vi "_UserDialog Choose Driver ReadMe Params.vi"(0 "VI Default Path":path, 1 "LV <help> directory?":bool, 2 "Documentable VI Path":path, 11 "error in (no error)":errorcluster) -> (4 "HTML File Path":path, 14 "Cancelled by User?":bool, 15 "error out":errorcluster)   [LabVIEW 2012]
uses:
  _Controls and TypeDefs/UserDialogStates.ctl
  <vilib>/Platform/browser.llb/Open URL in Default Browser (string).vi
panel:
  in  "www.labicom.net":bool
  in  "Help Button":bool
  in  "Revision History":string="REV 1.0, 16/07/2012\nModified by: Igor Titov, Geneva, CERN.\nOriginal release." caption="Provide detailed driver revision history including driver revision number, date of revision, and description of revision made to driver"
  in  "IsKnownIssues? chkBox":bool=TRUE
  in  "KnownIssues":string
  in  "SupportEmail":string="instrument.drivers@ni.com"
  in  "RequiredSoftware":string="[VISA 3.0 or later]"
  in  "CurrentRevisionDate":string="15/08/2012"
  in  "OriginalReleaseDate":string="15/08/2012"
  in  "DriverRevision":string="1.0"
  in  "FirmwareTested":string="[8-5-12]"
  in  "Interfaces":string="[GPIB, Serial, USB, Ethernet]"
  in  "ModelsTested":string="[33120A, 33220A]"
  in  "Languages":string="[LabVIEW]"
  in  "Models":string="[33120A, 33220A, 33250A]"
  in  "Manufacturer":string="[Agilent]"
  in  "IsCodeAvailable? Combo":string(combo)="Yes"
  in  "IsSupported? Combo":string(combo)="No"
  in  "IsCertified? Combo":string(combo)="No"
  in  "ProjectStyleCombo":string(combo)="(project-style)"
  in  "Disclaimer":string="[Disclaimer text]"
  in  "IsDisclaimer? chkBox":bool=TRUE
  in  "Cancel Button":bool
  in  "GenerateReadme_btn":bool
  in  "Patents":string="[Patents text]"
  in  "Trademarks":string="[Trademarks text]"
  in  "Copyright":string="[Copyright text]"
  in  "Support CommunityForums":string=" [link to community forums or NI Community page and expected response time]"
  in  "SupportEmail":string="[Support email address and expected response time]"
  in  "SupportTelephone":string="[Telephone number and hours of operation]"
  in  "AppUpgrader":string="[Developer Name, Developer e-mail, Developer certification level (if any), Organization]"
  in  "AppDeveloper":string="[Developer Name, Developer e-mail, Developer certification level (if any), Organization]"
  out "Product Short Name 12":string="[DriverIdentifier]" caption="Product Short Name"
  in  "IsDeveloper? chkBox":bool=TRUE
  in  "Installation Instructions":string[][](table)=[["[Step 1]"], ["[Step 2]"]]
  out "Product Short Name 2":string="[DriverIdentifier]" caption="Driver Identifier"
  in  "IsCopyright? chkBox":bool=TRUE
  in  "IsPatents? chkBox":bool=TRUE
  in  "IsTrademarks? chkBox":bool=TRUE
  in  "IsContactSupport? chkBox":bool=TRUE
  in  "IsInstallation? chkBox":bool=TRUE
  in  "Year":string="[Year]"
  in  "Month":string="[Month]"
  in  "Driver Identifier":string="[Driver Identifier]"
  in  "Next_btn":bool
  # "Instrument Driver Readme"
  # "To rate this instrument driver, go the the driver download page on the Instrument Driver Network."
  # "The readme contains the following main sections:"
  # "Overview"
  # "Required software"
  # "Revision History"
  # "1. Overview"
  # "Instrument Driver Technology: LabVIEW Plug and Play"
  # "Manufacturer:"
  # "Supported Language(s):"
  # "Supported Model(s):"
  # "Model(s) Tested:"
  # "Interface(s):"
  # "Firmware Revision(s) Tested:"
  # "Certified:"
  # "NI Supported:"
  # "Source Code Available:"
  # "Driver Revision:"
  # "Original Release Date:"
  # "Current Revision Date:"
  # "2. Installation (if applicable)"
  # "This section documents installation instructions for"
  # "Instrument Driver."
  # "New line here corresponds to new item in the list in HTML"
  # "3. Required Software"
  # "Some software components need to be installed before using this instrument driver. \nThe minimum versions of these components are listed below."
  # "Refer to the LabVIEW Help for more information about software requirements. \nYou access the LabVIEW Help by selecting Help»Search the LabVIEW Help."
  # "4. Known Issues (if applicable)"
  # "To report issues or provide feedback about this instrument driver, please send an email to"
  # "Include instrument functionality not supported by the driver or known issues as necessary."
  # "5. Revision History"
  # "The latest version of this and other LabVIEW and LabWindows/CVI instrument drivers can be downloaded \nat the Instrument Driver Network."
  # "6. Developer(s) of"
  # "Instrument Driver"
  # "(if applicable)"
  # "Step 2/2:\nConfigure VI Documentation Layout"
  # "This instrument driver was \ndeveloped by"
  # "Additional layout elements for LabVIEW help"
  # "This icon denotes a note, which alerts you\nto important information. You can add it\nby placing <_note_> into your text."
  # "Caution: place <_caution_> into your text"
  # "Last upgrade of this instrument driver was made by"
  # "Note: place <_note_> into your text"
  # "This icon denotes a caution, which \nadvises you of precautions to take to \navoid injury, data loss, or a system crash.\nYou can add it by placing <_caution_>\ninto your text."
  # "Mandatory Fields"
  # "7. Contact Support"
  # "Tip: place <_tip_> into your text"
  # "(if applicable)"
  # "You can contact our support staff by one of the following:"
  # "Windows"
  # "Platform: enclose platform name between\n<_platform_> and </_platform_> tags"
  # "Text in blue color denotes a specific \nplatform and indicates that the text \nfollowing it applies only to that platform.\nYou can add it enclosing platform name\nbetween <_platform_> and </_platform_>\ntags (e.g.: <_platform_>MacOS X</_platform_>)."
  # "Telephone:"
  # "bold"
  # "Text in bold: enclose such text between\n<B> and </B> tags"
  # "Email:"
  # "Community Forums:"
  # "Attention!"
  # "Caution Text: enclose such text between \n<_caution_text_> and </_caution_text_> tags"
  # "Bold text denotes items that you must \nselect or click on in the software, such as \nmenu items and dialog box options. \nBold text also denotes parameter names, \nemphasis, or an introduction to a key \nconcept. You can emphasize such text by \nenclosing in between <B> and </B> tags."
  # "vigods.com"
  # "Link: place relative path in place of '_path_' and\ntext in place of '_text_' and insert resulting string\nwherever you need: \n<a href=\"_path_\">_text_</a>"
  # "8. Copyright"
  # "monospace"
  # "Monospace: enclose such text between\n<_monospace_> and </_monospace_> tags"
  # "(if applicable)"
  # "9. Trademarks"
  # "(if applicable)"
  # "10. Patents"
  # "(if applicable)"
  # "11. Disclaimer"
  # "(if applicable)"
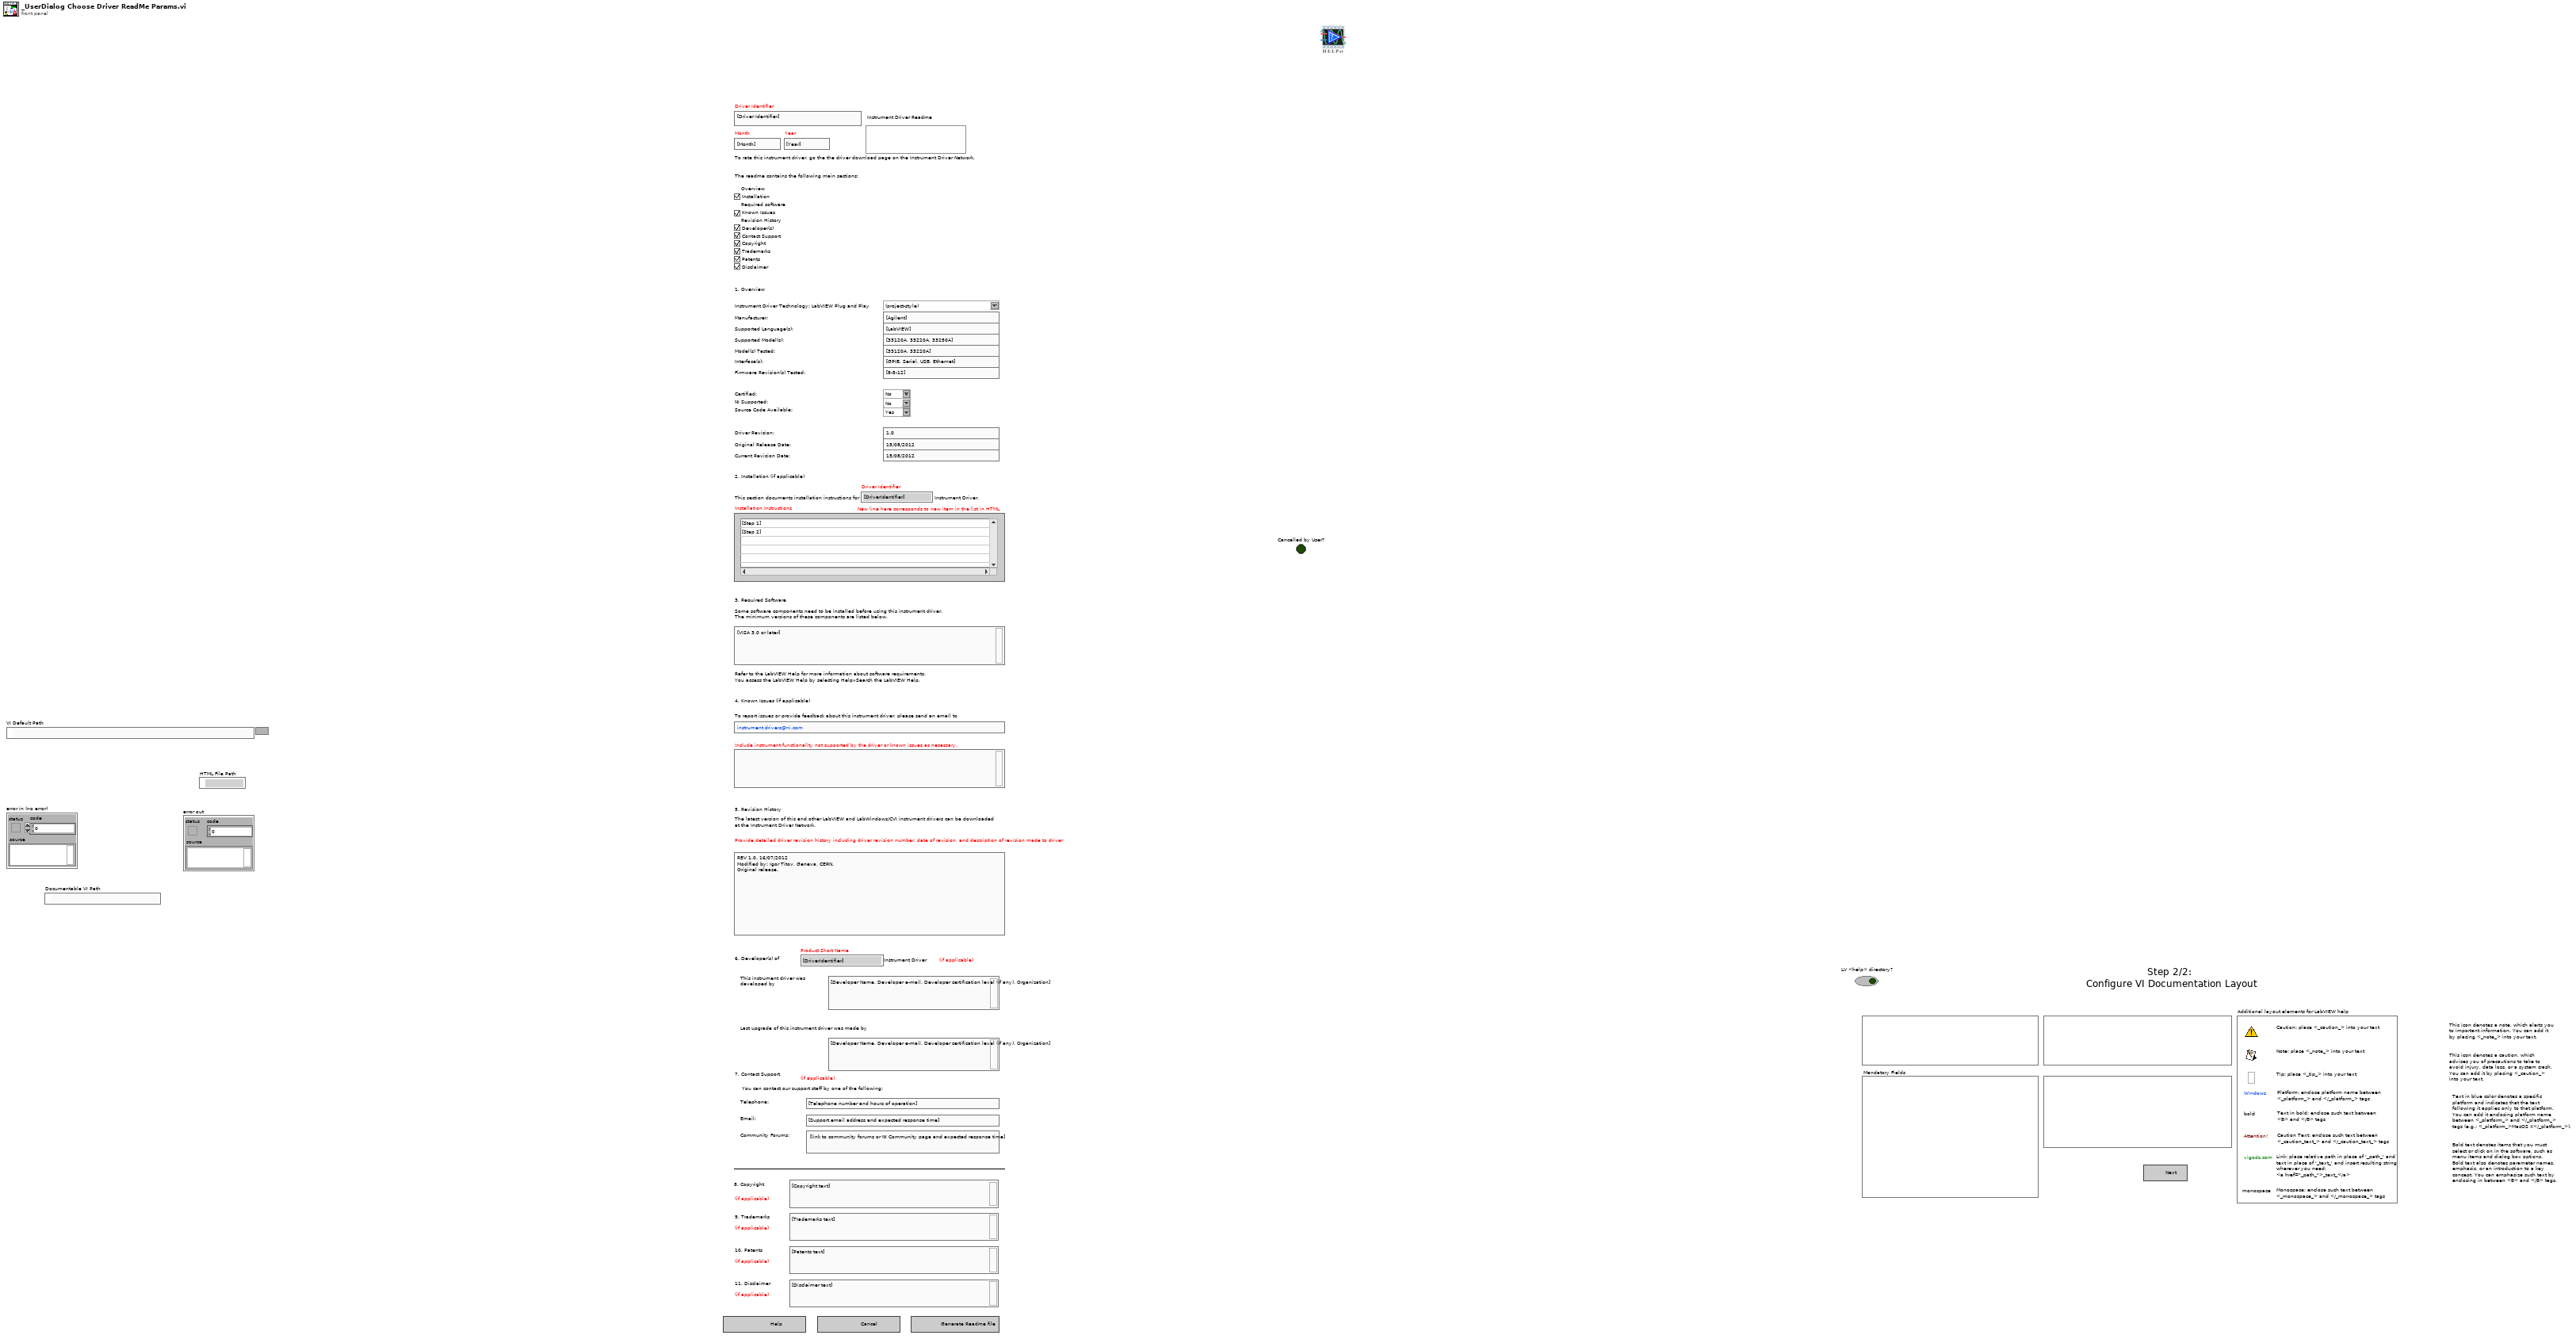
[diagram p1: front panel]
types:
  T1 = typedef "UserDialogStates.ctl" = enum16{"Overview", "Known Issues", "Choose parameters", "Update", "Choose HTML file path", "Choose Images directory path", "Decide if there is Context Help", "Choose help hierarchy", "Generate HTML", "Installation", "System Requirements", "Software Support", "Device Support", "Upgrade Issues", "New Features", "Fixed Issues", "Developer", "Contact Support", "Copyright", "Trademarks", "Patents", "Disclaimer", "Save", "Shutdown"}
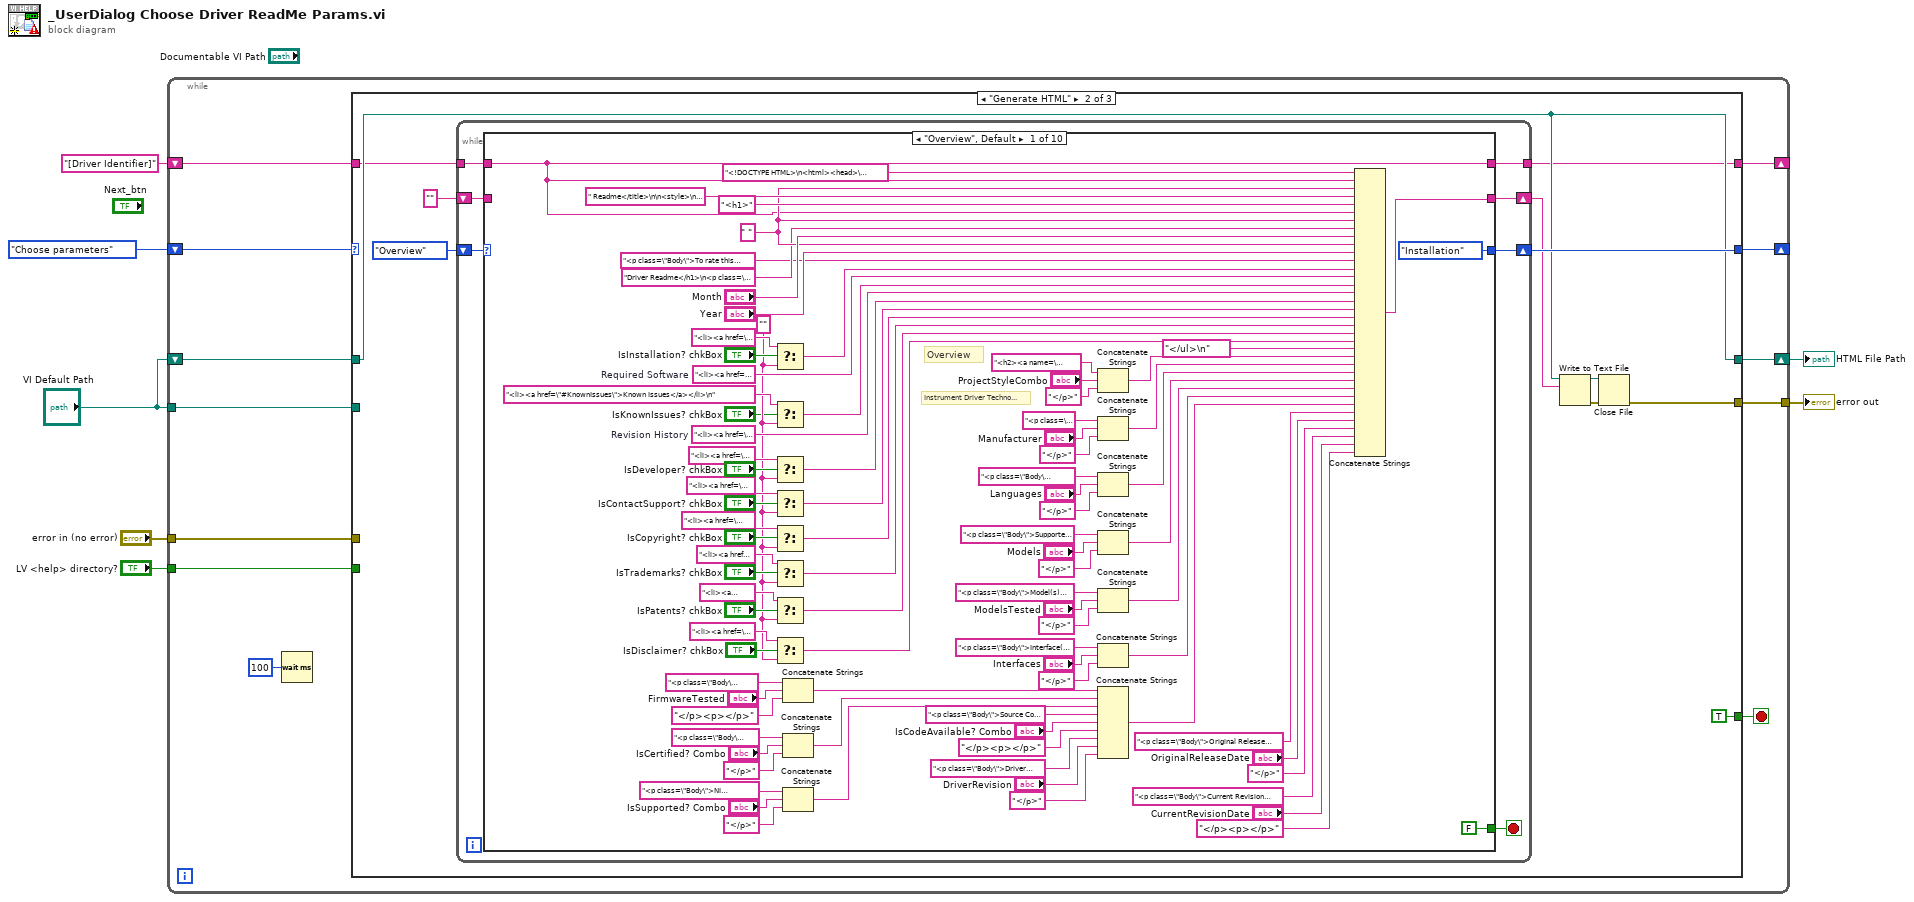
[diagram p0: block diagram]
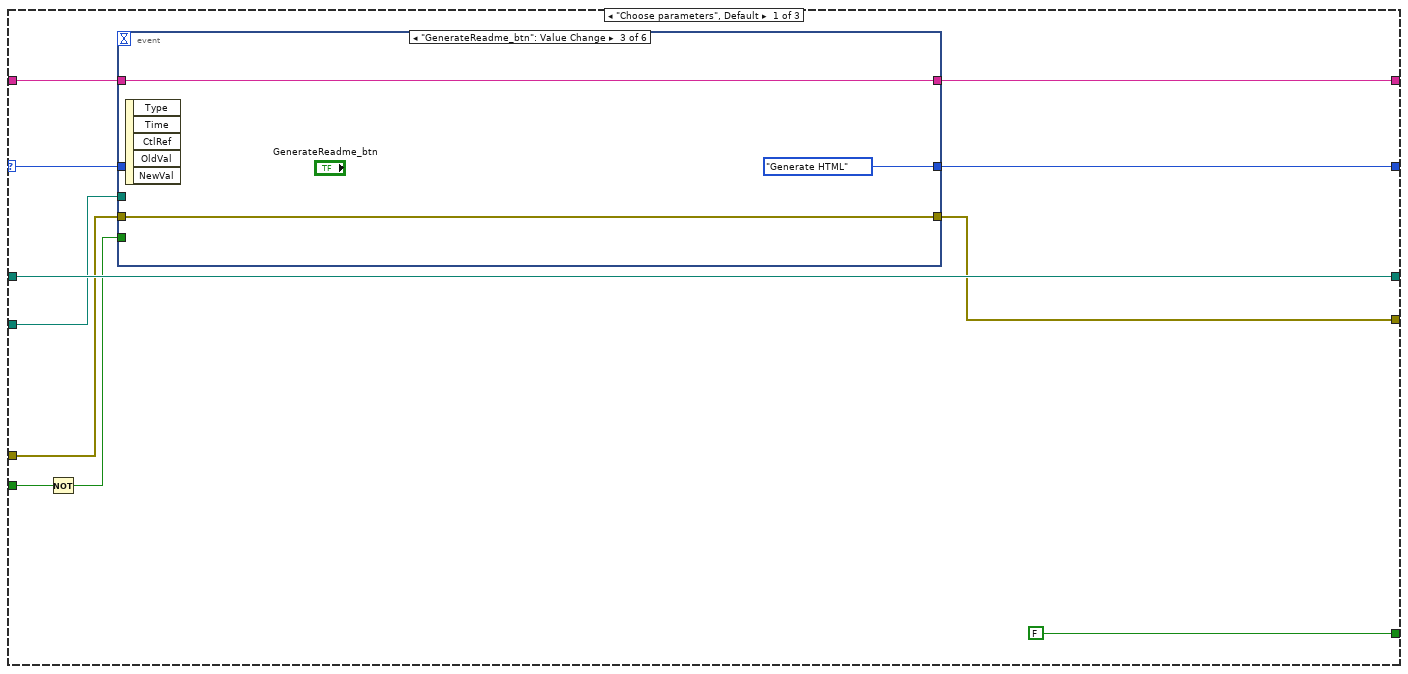
[diagram p2: hidden frame]
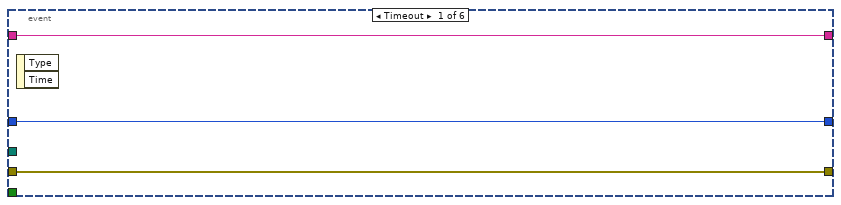
[diagram p3: hidden frame]
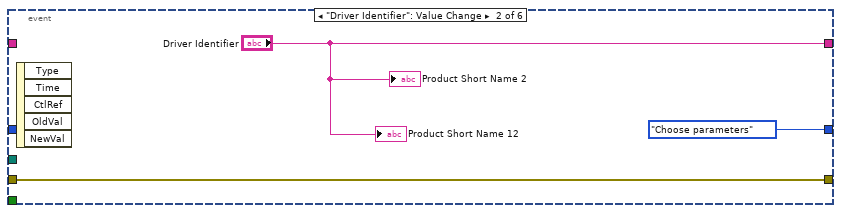
[diagram p4: hidden frame]
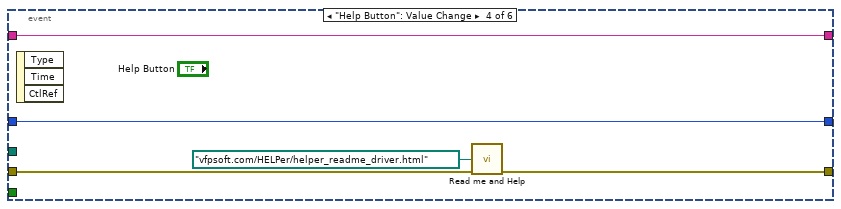
[diagram p5: hidden frame]
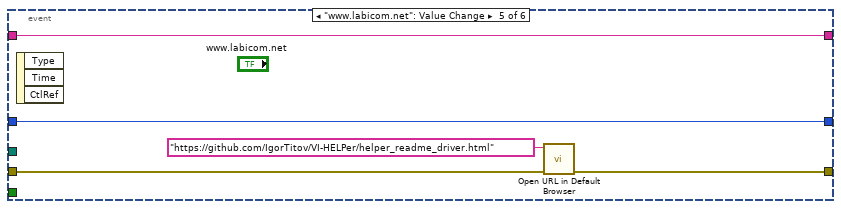
[diagram p6: hidden frame]
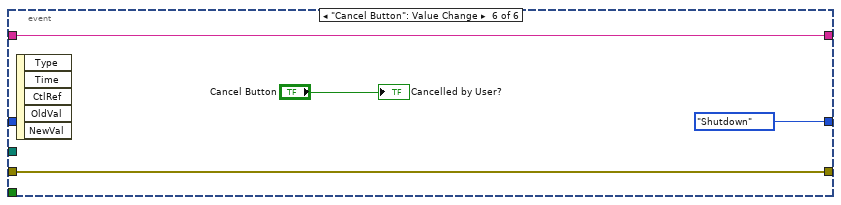
[diagram p7: hidden frame]
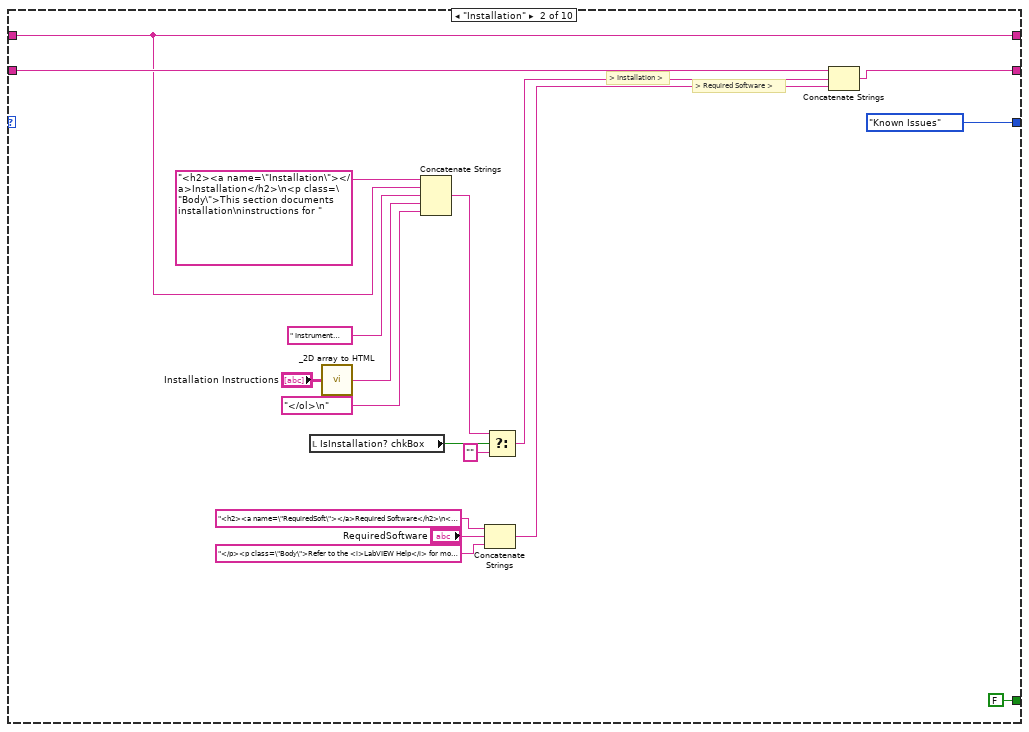
[diagram p8: hidden frame]
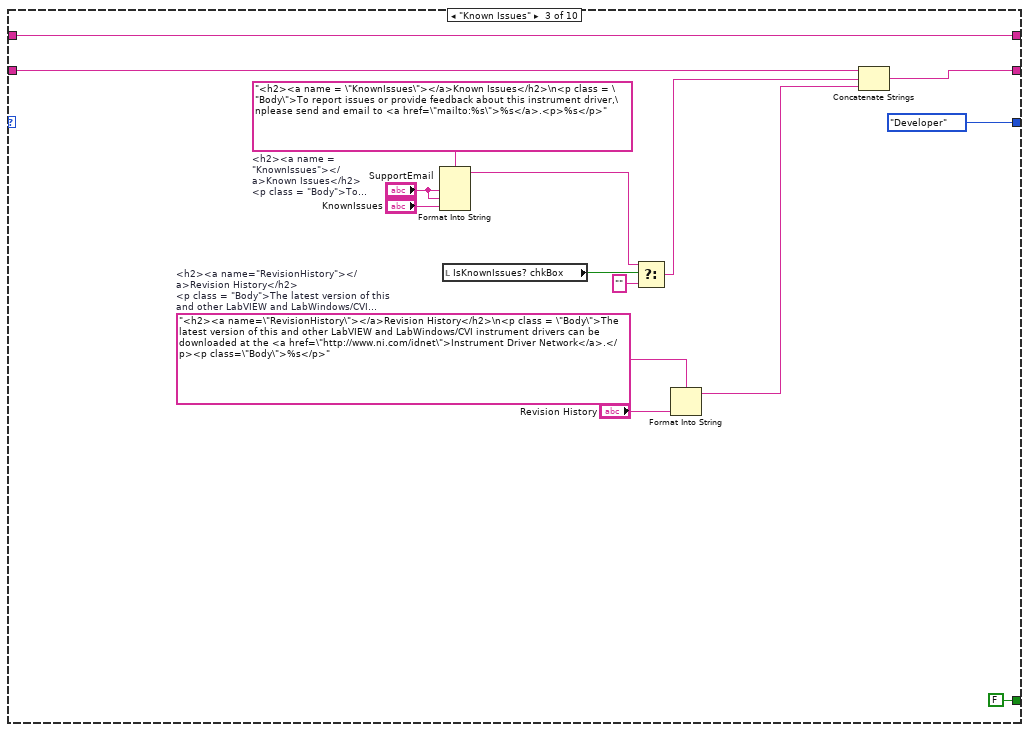
[diagram p9: hidden frame]
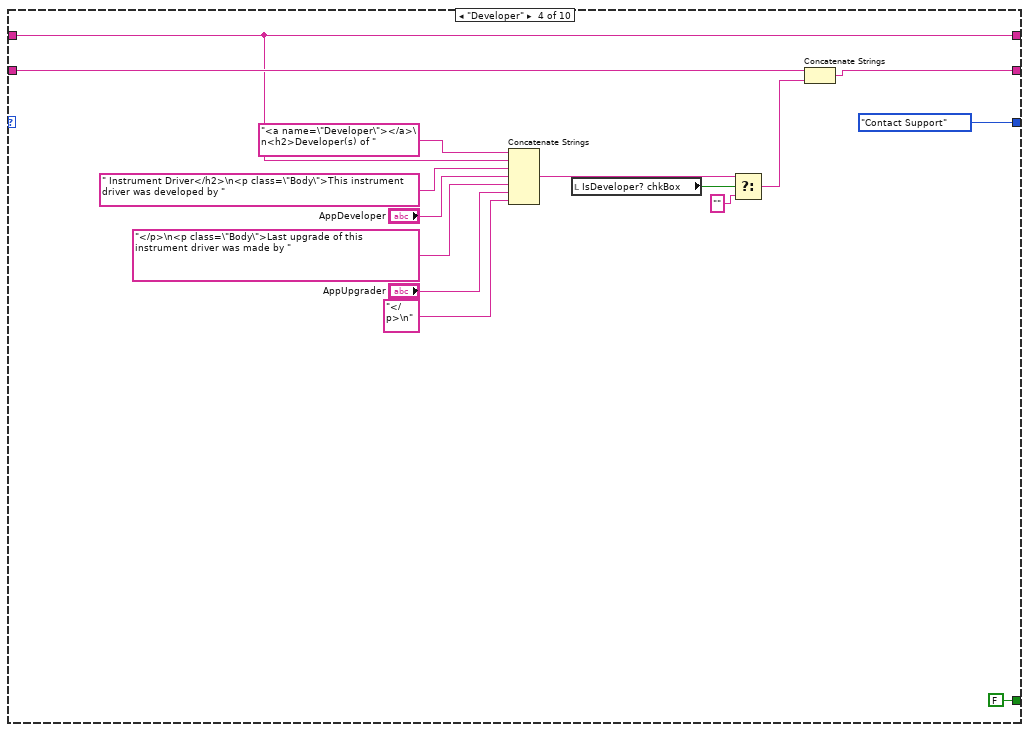
[diagram p10: hidden frame]
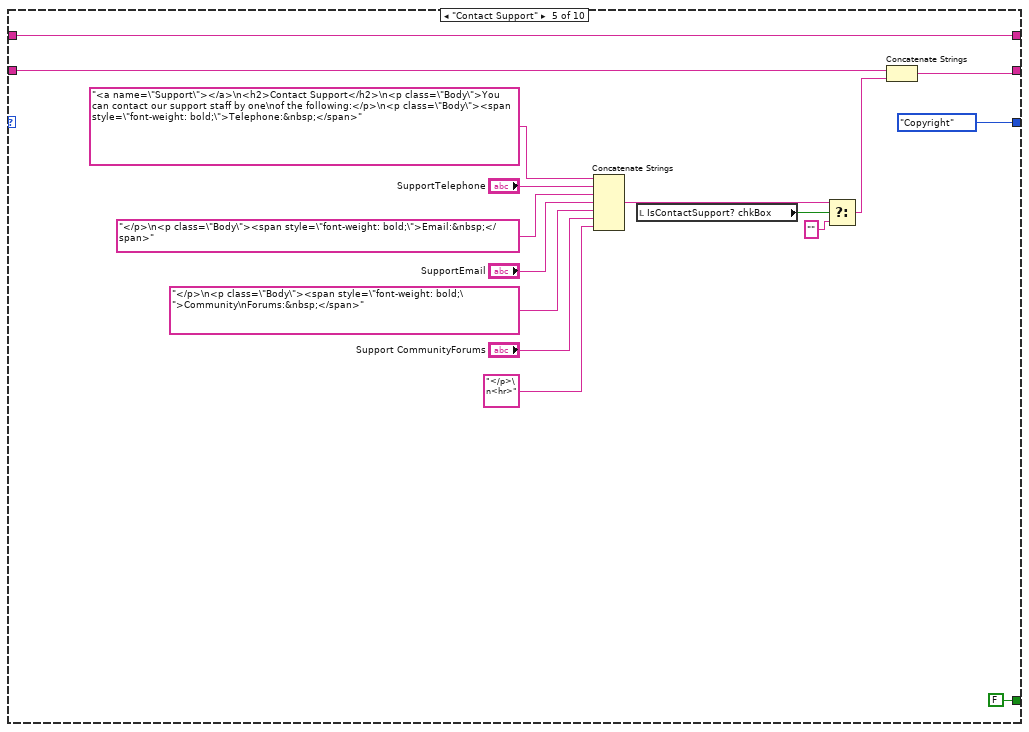
[diagram p11: hidden frame]
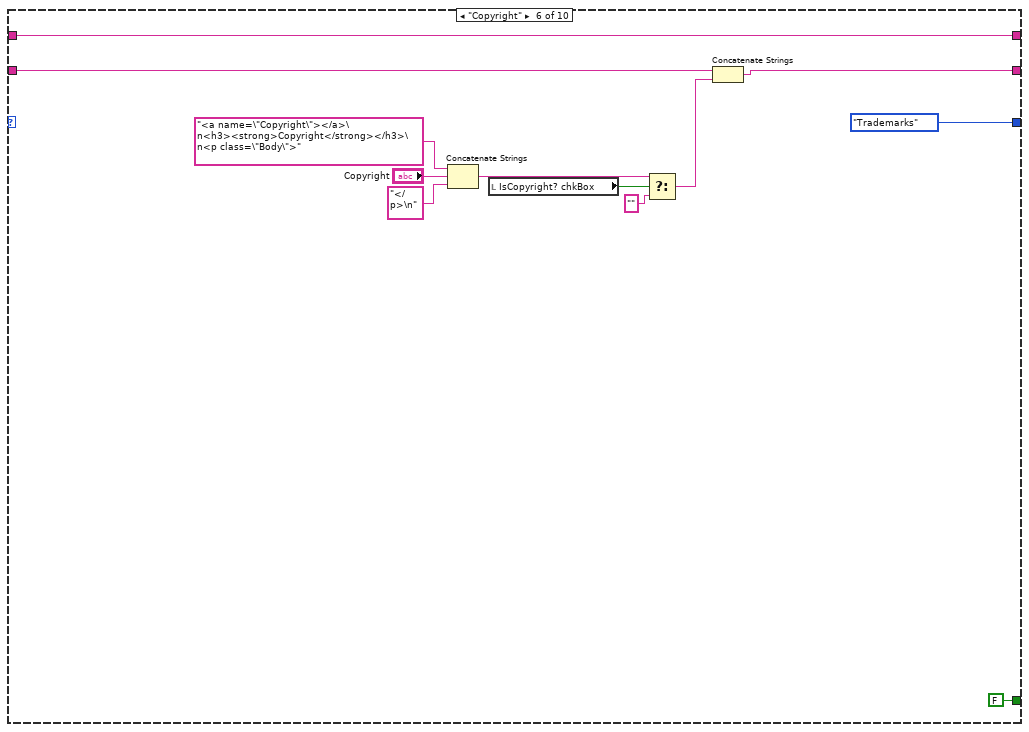
[diagram p12: hidden frame]
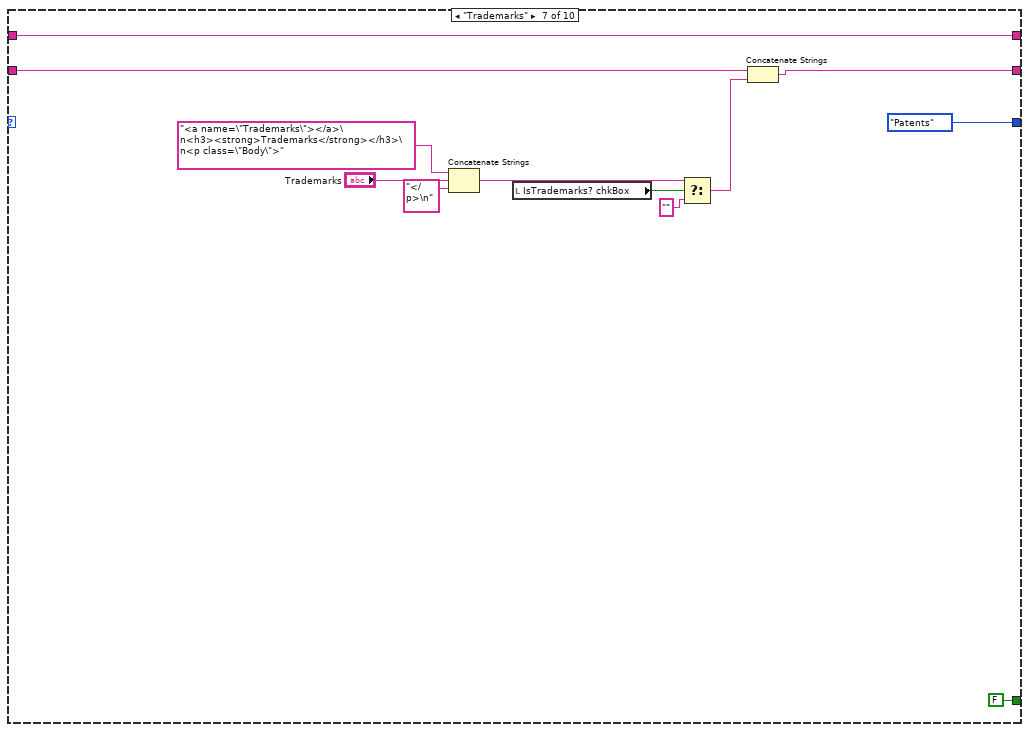
[diagram p13: hidden frame]
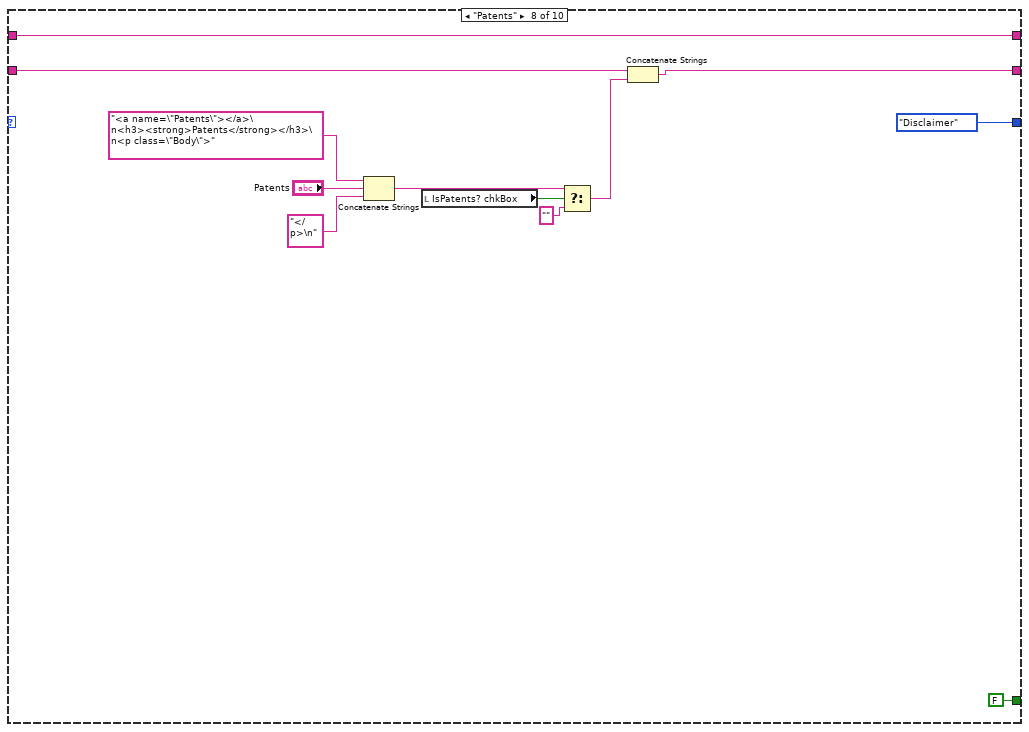
[diagram p14: hidden frame]
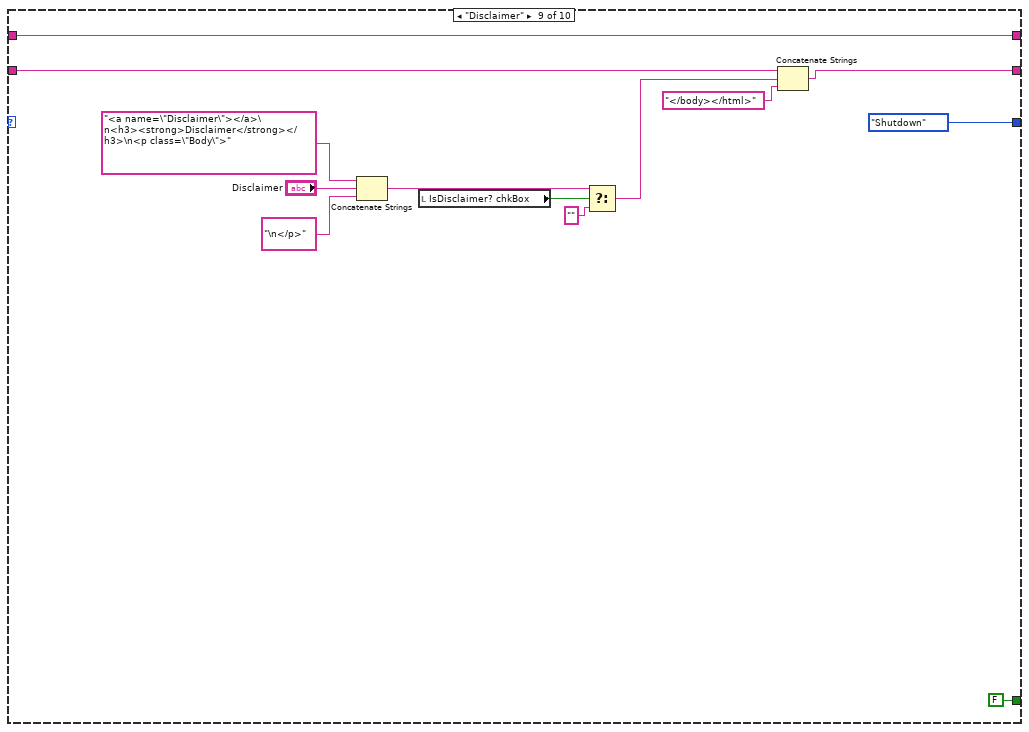
[diagram p15: hidden frame]
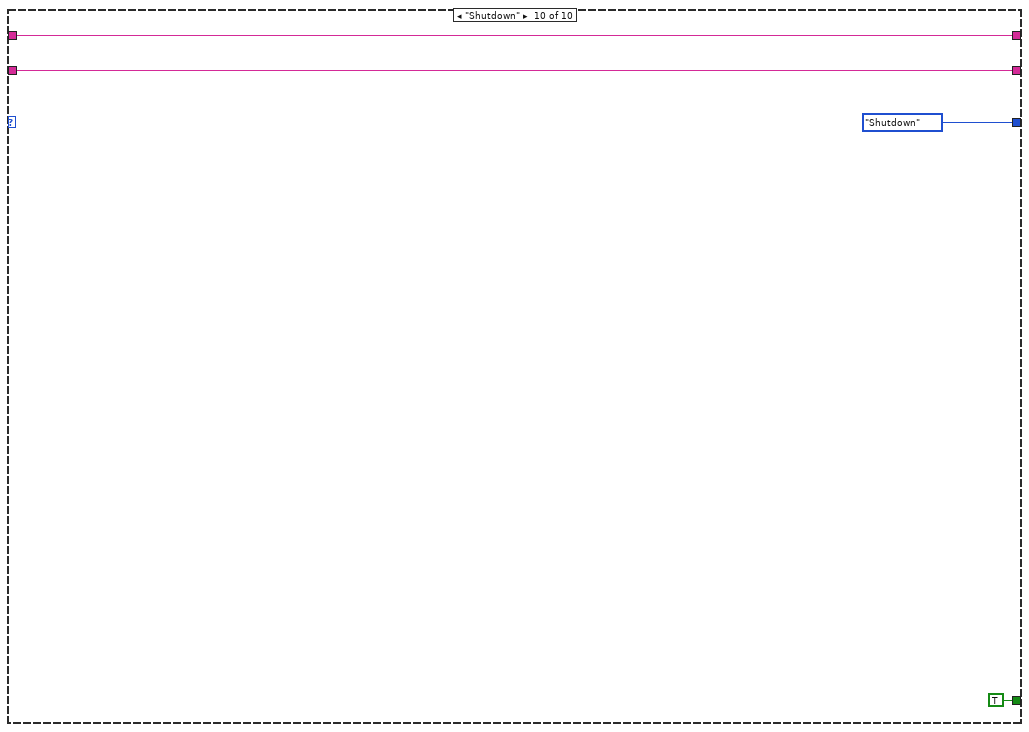
[diagram p16: hidden frame]
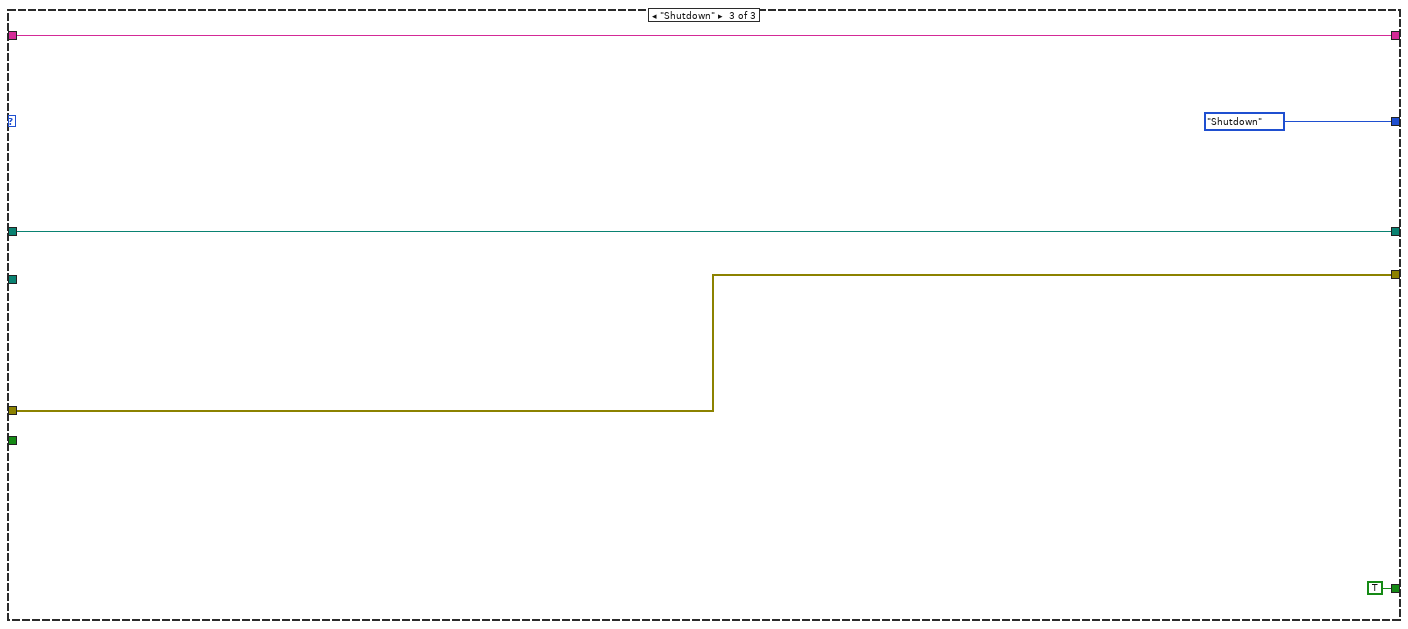
[diagram p17: hidden frame]
diagram:
  n1 = while {
    shift-right: [w16] -> _
    shift-left: UserDialogStates."Choose parameters" ("UserDialogSteps") -> [w17]
    tunnel: "VI Default Path" -> [w15]
    shift-right: [w14] -> w6
    shift-left: "VI Default Path" -> [w13]
    tunnel: "LV <help> directory?" -> [w8]
    tunnel: "error in (no error)" -> [w12]
    shift-right: [w11] -> _
    shift-left: "[Driver Identifier]" ("Driver Identifier") -> [w10]
    tunnel: [w9] -> w1
    stop <- w19 stop-if-true
    n2 = Wait (ms)(milliseconds to wait=u32 100) -> ()  [unwired: 1 out]
    n3 = case shown="\"Generate HTML\"" w17 {
      selector: w17 -> [w29 _ _]
      tunnel: [FALSE TRUE TRUE] -> w19
      tunnel: [w28 w63 UserDialogStates."Shutdown" ("UserDialogSteps")] -> w16
      tunnel: w15 -> [w25 _ _]
      tunnel: [w27 w61 w282] -> w14
      tunnel: w13 -> [w27 w61 w282]
      tunnel: w8 -> [w26 _ _]
      tunnel: w12 -> [w23 _ w278]
      tunnel: w10 -> [w22 w57 w280]
      tunnel: [w21 w56 w280] -> w11
      tunnel: [w20 w54 w278] -> w9
      frame "Choose parameters", Default {
        n4 = Not(x=w26) -> (.not. x?=w24:bool)
        n5 = event shown="[2] \"GenerateReadme_btn\": Value Change" {
          selector: _ -> [_ _ _ _ _ _]
          dyn-events: _ -> [_ _ _ _ _ _]
          timeout: _ -> [_ _ _ _ _ _]
          tunnel: w29 -> [w33 _ _ w44 w45 _]
          tunnel: [w33 UserDialogStates."Choose parameters" ("UserDialogSteps") UserDialogStates."Generate HTML" ("UserDialogSteps") w44 w45 UserDialogStates."Shutdown" ("UserDialogSteps")] -> w28
          tunnel: w25 -> [_ _ _ _ _ _]
          tunnel: w24 -> [_ _ _ _ _ _]
          tunnel: w23 -> [w31 w35 w38 w42 w48 w51]
          tunnel: w22 -> [w32 _ w39 w43 w46 w52]
          tunnel: [w32 "Driver Identifier" w39 w43 w46 w52] -> w21
          tunnel: [w31 w35 w38 w41 w47 w51] -> w20
          event Timeout {
            n6 = event-data() -> ()  [unwired: 1 in, 2 out]
          }
          event "Driver Identifier": Value Change {
            n7 = event-data() -> ()  [unwired: 1 in, 5 out]
            "Product Short Name 2" <- "Driver Identifier"
            "Product Short Name 12" <- "Driver Identifier"
          }
          event "GenerateReadme_btn": Value Change {
            n8 = event-data() -> ()  [unwired: 1 in, 5 out]
          }
          event "Help Button": Value Change {
            n9 = event-data() -> ()  [unwired: 1 in, 3 out]
            n10 = call "Read me and Help.vi"("path"=path "vfpsoft.com/HELPer/helper_readme_driver.html", "error in"=w42) -> ("error out"=w41:errorcluster)  [unwired: 13 in]
          }
          event "www.labicom.net": Value Change {
            n11 = event-data() -> ()  [unwired: 1 in, 3 out]
            n12 = call-poly <vilib>:"Open URL in Default Browser.vi"("error in (no error)"=w48, "URL"="https://github.com/IgorTitov/VI-HELPer/helper_readme_driver.html") -> ("error out"=w47:errorcluster)  [unwired: 4 in, 1 out]
          }
          event "Cancel Button": Value Change {
            n13 = event-data() -> ()  [unwired: 1 in, 5 out]
            "Cancelled by User?" <- "Cancel Button"
          }
        }
      }
      frame "Generate HTML" {
        n14 = while {
          shift-right: [w70] -> w63
          shift-left: UserDialogStates."Overview" ("UserDialogSteps") -> [w71]
          shift-right: [w68] -> w60
          shift-left: "" -> [w69]
          tunnel: w57 -> [w66]
          tunnel: [w65] -> w56
          stop <- w67 stop-if-true
          n15 = case shown="\"Overview\", Default" w71 {
            tunnel: [UserDialogStates."Installation" ("UserDialogSteps") UserDialogStates."Known Issues" ("UserDialogSteps") UserDialogStates."Developer" ("UserDialogSteps") UserDialogStates."Contact Support" ("UserDialogSteps") UserDialogStates."Copyright" ("UserDialogSteps") UserDialogStates."Trademarks" ("UserDialogSteps") UserDialogStates."Patents" ("UserDialogSteps") UserDialogStates."Disclaimer" ("UserDialogSteps") UserDialogStates."Shutdown" ("UserDialogSteps") UserDialogStates."Shutdown" ("UserDialogSteps")] -> w70
            tunnel: w69 -> [_ w169 w191 w206 w221 w233 w245 w257 w269 w276]
            tunnel: [w124 w167 w190 w205 w220 w232 w244 w256 w271 w276] -> w68
            tunnel: [FALSE FALSE FALSE FALSE FALSE FALSE FALSE FALSE FALSE TRUE] -> w67
            tunnel: w66 -> [w73 w162 w187 w195 w210 w226 w238 w250 w262 w275]
            tunnel: [w73 w162 w187 w195 w210 w226 w238 w250 w262 w275] -> w65
            frame "Overview", Default {
              w126 = "<li><a href=\"#RevisionHistory\">Revision History</a></li>\n"  # Revision History
              w127 = "<li><a href=\"#RequiredSoft\">Required Software</a></li>\n"  # Required Software
              w125 = ""
              w130 = " " ("string")
              # "Instrument Driver Techno..."
              # "Overview"
              n16 = Select(t="<li><a href=\"#Installation\">Installation</a></li>\n", s="IsInstallation? chkBox", f=w125) -> (s? t:f=w156:string)
              n17 = Select(t="<li><a href=\"#KnownIssues\">Known Issues</a></li>\n", s="IsKnownIssues? chkBox", f=w125) -> (s? t:f=w154:string)
              n18 = Select(t="<li><a href=\"#Developer\">Developer(s)</a></li>", s="IsDeveloper? chkBox", f=w125) -> (s? t:f=w152:string)
              n19 = Select(t="<li><a href=\"#Support\">Contact Support</a></li>\n", s="IsContactSupport? chkBox", f=w125) -> (s? t:f=w149:string)
              n20 = Select(t="<li><a href=\"#Copyright\">Copyright</a></li>\n", s="IsCopyright? chkBox", f=w125) -> (s? t:f=w145:string)
              n21 = Select(t="<li><a href=\"#Trademarks\">Trademarks</a></li>\n", s="IsTrademarks? chkBox", f=w125) -> (s? t:f=w139:string)
              n22 = Select(t="<li><a href=\"#Patents\">Patents</a></li>\n", s="IsPatents? chkBox", f=w125) -> (s? t:f=w138:string)
              n23 = Select(t="<li><a href=\"#Disclaimer\">Disclaimer</a></li>\n", s="IsDisclaimer? chkBox", f=w125) -> (s? t:f=w135:string)
              n24 = Concatenate Strings("<p class=\"Body\">Firmware Revision(s) Tested: ", "FirmwareTested", "</p><p></p>") -> (w88:string)
              n25 = Concatenate Strings("<p class=\"Body\">Certified: ", "IsCertified? Combo", "</p>") -> (w87:string)
              n26 = Concatenate Strings("<p class=\"Body\">NI Supported: ", "IsSupported? Combo", "</p>") -> (w86:string)
              n27 = Concatenate Strings("<h2><a name=\"Overview\"></a>Overview</h2>\n<p class=\"Body\">Instrument Driver Technology: LabVIEW Plug and Play ", "ProjectStyleCombo", "</p>") -> (w121:string)
              n28 = Concatenate Strings("<p class=\"Body\">Manufacturer: ", "Manufacturer", "</p>") -> (w117:string)
              n29 = Concatenate Strings("<p class=\"Body\">Supported Language(s): ", "Languages", "</p>") -> (w113:string)
              n30 = Concatenate Strings("<p class=\"Body\">Supported Model(s): ", "Models", "</p>") -> (w109:string)
              n31 = Concatenate Strings("<p class=\"Body\">Model(s) Tested: ", "ModelsTested", "</p>") -> (w105:string)
              n32 = Concatenate Strings("<p class=\"Body\">Interface(s): ", "Interfaces", "</p>") -> (w101:string)
              n33 = Concatenate Strings(w88, w87, w86, "<p class=\"Body\">Source Code Available: ", "IsCodeAvailable? Combo", "</p><p></p>", "<p class=\"Body\">Driver Revision: ", "DriverRevision", "</p>") -> (w85:string)
              n34 = Concatenate Strings("<!DOCTYPE HTML>\n<html><head>\n<meta http-equiv=\"Content-Type\" content=\"text/html; charset=ISO-8859-1\">\n<META NAME=\"GENERATOR\" CONTENT=\"HELPer - VI Documentation Toolkit from https://github.com/IgorTitov/VI-HELPer\">\n<script>\nfunction Link(URL)\n{\nwindow.location = URL;\n}\n</script>\n<meta http-equiv=\"Content-Type\" content=\"text/html; charset=ISO-8859-1\"><title>", w73, w130, " Readme</title>\n\n<style>\n/***************************************************/\n/* MINIMAL STYLES */\n/* The following section defines styles that every HTML Help project should\nneed. */\n/* The default style of P is red to alert you that you need to apply a style\nclass, such as Body. */\nP { margin-top:6.00pt; margin-bottom:6.00pt; font-family:Verdana; font-size:8pt;\ncolor: #FF0000; }\nBR { font-size:4.00pt; }\n/* Use H1 for all topic headings. */\nH1 { margin-top:3.00pt; margin-bottom:3.00pt; font-family:Verdana;\nfont-size:12pt; font-weight:bold; }\n/* Use H2 for second-level headings. */\nH2 { margin-top:9.00pt; margin-bottom:3.00pt; font-family:Verdana;\nfont-size:10pt; font-weight:bold; }\n/* Use H3 for third-level headings. */\nH3 { margin-top:6.00pt; margin-bottom:3.00pt; font-family:Verdana;\nfont-size:8pt; font-weight:bold; }\n/* Use H4 for fourth-level headings. */\nH4 { margin-top:3.00pt; margin-bottom:3.00pt; font-family:Verdana;\nfont-size:8pt; font-weight:bold; }\n/* H5 and H6 have the same definition as H4 because you should not need this\nlevel of heading in one topic. If you need to use H5 or H6, consider breaking up\nyour topic into more than one topic. */\nH5 { margin-top:3.00pt; margin-bottom:3.00pt; font-family:Verdana;\nfont-size:8pt; font-weight:bold; }\nH6 { margin-top:3.00pt; margin-bottom:3.00pt; font-family:Verdana;\nfont-size:8pt; font-weight:bold; }\n/* Use the Body style class for normal paragraphs. */\nP.Body { margin-top:6.00pt; margin-bottom:6.00pt; font-family:Verdana;\nfont-size:8pt; color:black; }\n/* Use the Anchor style class for graphic references on a line by themselves. */\nP.Anchor { margin-top:6.00pt; margin-bottom:6.00pt; font-family:Verdana;\nfont-size:10pt; color:black; }\n/* Use the Indent style classes to indent a paragraph. If you need to indent\ntext below a list item, use <br><br> to start the new paragraph within the same\nset of <li></li> tags. If you need to indent a list within another list, nest\nthe indented list within the first list's set of <ol></ol> or <ul></ul> tags. */\nP.Indent1 { margin-left:12.00pt; margin-top:6.00pt; margin-bottom:3.00pt;\nfont-family:Verdana; font-size:8pt; color:black; }\nP.Indent2 { margin-left:24.00pt; margin-top:6.00pt; margin-bottom:3.00pt;\nfont-family:Verdana; font-size:8pt; color:black; }\nP.Indent3 { margin-left:36.00pt; margin-top:6.00pt; margin-bottom:3.00pt;\nfont-family:Verdana; font-size:8pt; color:black; }\n/* Use the LI style for all list items. */\nLI { margin-top:3.00pt; margin-bottom:3.00pt; font-family:Verdana;\nfont-size:8pt; color:black; }\n/* Use the OL style for numbered lists. You do not have to type the number for\neach list item in a numbered list. */\nOL { margin-left:18.00pt; margin-top:3.00pt; margin-bottom:3.00pt;\ntext-indent:0pt; font-family:Verdana; font-size:8pt; color:black;\nlist-style-type: decimal; }\n/* Use the EquationNum style class for numbered lists of equations. You do not\nhave to type the number for each list item in a numbered list. */\nOL.EquationNum { margin-left:36.00pt; margin-top:3.00pt; margin-bottom:3.00pt;\ntext-indent:0pt; font-family:Verdana; font-size:8pt; color:black;\nlist-style-type: decimal; }\n/* Use the List-abc style class for lettered lists. You do not have to type the\nletter for each list item in a lettered list. */\nOL.List-abc { margin-left:18.00pt; margin-top:3.00pt; margin-bottom:3.00pt;\ntext-indent:0pt; font-family:Verdana; font-size:8pt; color:black;\nlist-style-type:lower-alpha; }\n/* Use the UL style for bulleted lists. You do not have to type the bullet for\neach list item in a bulleted list. */\nUL { margin-left:12.00pt; text-indent:0pt; margin-top:3.00pt;\nmargin-bottom:3.00pt; font-family:Verdana; font-size:8pt; color:black;\nlist-style-type: disc; }\n/* Use the List-Box style class for bulleted lists with boxes instead of\nbullets. You do not have to type the box for each list item in a box list. */\nUL.List-Box { margin-left:12.00pt; margin-top:3.00pt; margin-bottom:3.00pt;\ntext-indent:0pt; font-family:Verdana; font-size:8pt; color:black;\nlist-style-type: square; }\n/* Use the List-Diamond style class for bulleted lists with diamonds instead of\nbullets. You do not have to type the diamond for each list item in a diamond\nlist. */\nUL.List-Diamond { margin-left:12.00pt; margin-top:3.00pt; margin-bottom:3.00pt;\ntext-indent:0pt; font-family:Verdana; font-size:8pt; color:black;\nlist-style-image:url(diamond.gif); }\n/* Use the List-Hyphen style class for bulleted lists with hyphens instead of\nbullets. You do not have to type the hyphen for each list item in a hyphen list.\n*/\nUL.List-Hyphen { margin-left:12.00pt; margin-top:3.00pt; margin-bottom:3.00pt;\ntext-indent:0pt; font-family:Verdana; font-size:8pt; color:black;\nlist-style-image:url(hyphen.gif); }\n/* Use the Borderless style class for tables that do not need borders, such as\nfor 2-column or 3-column lists with no headings. */\nTable.Borderless { border:none; }\n/* Use the Bordered style class for tables that need borders. */\nTable.Bordered { border-width: 1pt; border-style: solid; border-color: black;\nborder-collapse: collapse; }\n/* Use the Borderless-Wide style class for tables that do not need borders and\nthat you want to stretch to fill the entire topic width. */\nTable.Borderless-Wide { border:none; width:100%; }\n/* Use the Bordered-Wide style class for tables that need borders and that you\nwant to stretch to fill the entire topic width. */\nTable.Bordered-Wide { border-width: 1pt; border-style: solid; border-color:\nblack; width:100%; border-collapse: collapse; }\n/* Use the TD style for table cells in Borderless or Borderless-Wide tables. */\nTD { font-family:Verdana; font-size:8pt; color:black; vertical-align:top;\npadding:3px; }\n/* Use the Bordered style class for table cells in Bordered or Bordered-Wide\ntables. */\nTD.Bordered { font-family:Verdana; font-size:8pt; color:black;\nvertical-align:top; border-width: 1pt; border-style: solid; border-color: black;\n}\n/* Use the Icon style class for table cells that contain note, caution, warning,\nor tip icons, or LabVIEW datatype terminals. */\nTD.Icon { width:40px; vertical-align:top; }\n/* Use the Table-cell-8pt style class for table cells in tables that contain a\nlot of information and need smaller text to fit it all on one screen to prevent\na horizontal scroll bar from appearing. */\nTD.Table-cell-8pt { font-family:Verdana; font-size:7pt; color:black; }\n/* Use the TH style for table heading cells in Borderless or Borderless-Wide\ntables. */\nTH { font-family:Verdana; font-size:8pt; color:black; font-weight:bold;\npadding:3px; }\n/* Use the Bordered style class for table heading cells in Bordered or\nBordered-Wide tables. */\nTH.Bordered { font-family:Verdana; font-size:8pt; color:black; font-weight:bold;\nborder-width: 1pt; border-style: solid; border-color: black; }\n/* Use the Table-cell-8pt style class for table heading cells in tables that\ncontain a lot of information and need smaller text to fit it all on one screen\nto prevent a horizontal scroll bar from appearing. */\nTH.Table-Head-8pt { font-family:Verdana; font-size:7pt; color:black;\nfont-weight:bold; }\n/* Use the Left-Align style class for table heading cells that you want to left\nalign instead of center align. */\nTH.Left-Align { font-family:Verdana; font-size:8pt; color:black;\nfont-weight:bold; padding:3px; text-align:left; }\n/***************************************************/\n/* CHARACTER FORMATS */\n/* The following section defines character formats that every HTML Help project\nshould need. */\n/* Use the Dark-Red format for warnings or cautions. */\n#Dark-Red { color: #800000 }\n/* Use the Monospace format for code or syntax examples. */\n#Monospace { font-family: Courier New; font-size: 8pt; }\n/* Use the Monospace-Bold format for messages and responses that the computer\nautomatically prints to the screen. */\n#Monospace-Bold { font-family: Courier New; font-size: 8pt; font-weight: bold; }\n/* Use the Monospace-Italic format to denote text that is a placeholder for a\nword or value that the user must supply. */\n#Monospace-Italic { font-family: Courier New; font-size: 8pt; font-style:\nitalic; }\n/* Use the Platform format to denote a specific platform. */\n#Platform { color: #0000FF; font-weight: bold; }\n/* Use the Symbol format for characters not in the Verdana character set. Use\nthis format sparingly. When possible, you should use the correct ASCII code for\nthe symbol or use a graphic to recreate the symbol. */\n#Symbol { font-family: Symbol; font-size: 8pt; }\n/* CHARACTER FORMATS Updated to conform with the CSE HTML Validator Pro */\n/* The following section defines character formats that every HTML Help project\nshould need. */\n/* Use the Dark-Red format for warnings or cautions. */\n.Dark-Red { color: #800000 }\n/* Use the Monospace format for code or syntax examples. */\n.Monospace { font-family: Courier New; font-size: 8pt; }\n/* Use the Monospace-Bold format for messages and responses that the computer\nautomatically prints to the screen. */\n.Monospace-Bold { font-family: Courier New; font-size: 8pt; font-weight: bold; }\n/* Use the Monospace-Italic format to denote text that is a placeholder for a\nword or value that the user must supply. */\n.Monospace-Italic { font-family: Courier New; font-size: 8pt; font-style:\nitalic; }\n/* Use the Platform format to denote a specific platform. */\n.Platform { color: #0000FF; font-weight: bold; }\n/* Use the Symbol format for characters not in the Verdana character set. Use\nthis format sparingly. When possible, you should use the correct ASCII code for\nthe symbol or use a graphic to recreate the symbol. */\n.Symbol { font-family: Symbol; font-size: 8pt; }\n/* Use the Red-text format to call attention to text that needs information\nadded or edited by techcomm */\n.Red-text {color: #FF0000;}\n/* Use the Green-Underline format for the green defintion in the conventions\ntopic */\n.Green-Underline {color: #007700; text-decoration : underline;}\n/* Use the glossButton format for the glossary buttons used in the glossary\ntopic */\n.glossButton { font-family:Verdana, sans-serif; font-size:12px; color:black; }\n/* Use for text sections and hyphenated words that should not break at line\nwraps */\nspan.nobreak{white-space:nowrap}\n/* The following styles define the color of links. */\na:link { color: #007700 }\na:hover { color: #FF0000 }\na:active { color: #FF0000 }\na:visited { color: #7F007F }\n/***************************************************/\n/* ACTIVITY STYLES */\n/* The following section defines styles that only tutorial-style HTML Help\nprojects should need. */\n/* Use the Activity-Objective style class for the objective at the beginning of\nan activity topic. */\nH3.Activity-Objective { color: #800000; }\n/***************************************************/\n/* CODE STYLES */\n/* The following section defines styles that you need to format entire sections\nof code or syntax examples. If you have just a few words you need to format as a\ncode or syntax example, use the Monospace character format. */\nP.Code { margin-top:3.00pt; margin-bottom:0.00pt; font-family:Courier New;\nfont-size:8pt; color:black; }\nP.Code1 { margin-left:12.00pt; margin-top:3.00pt; margin-bottom:0.00pt;\nfont-family:Courier New; font-size:8pt; color:black; }\nP.Code2 { margin-left:24.00pt; margin-top:3.00pt; margin-bottom:0.00pt;\nfont-family:Courier New; font-size:8pt; color:black; }\nP.Code3 { margin-left:36.00pt; margin-top:3.00pt; margin-bottom:0.00pt;\nfont-family:Courier New; font-size:8pt; color:black; }\n/***************************************************/\n/* FUNCTION STYLES */\n/* The following section defines styles that you might need to format function\nreference help. */\nP.F-VI-Code4 { margin-left:48.00pt; margin-top:3.00pt; margin-bottom:0.00pt;\nfont-family:Courier New; font-size:8pt; color:black; }\nP.F-VI-Code5 { margin-left:60.00pt; margin-top:3.00pt; margin-bottom:0.00pt;\nfont-family:Courier New; font-size:8pt; color:black; }\nP.F-VI-Equation { margin-top:9.00pt; margin-bottom:9.00pt; font-family:Verdana;\nfont-size:8pt; color:black; }\nOL.F-VI-EquationNum { margin-top:3.00pt; margin-bottom:3.00pt; text-indent:0pt;\nfont-family:Verdana; font-size:8pt; color:black; list-style-type: decimal; }\nCITE.expandspot { font-style : normal;\ncolor : green;\ncursor: hand;}\n.mvd-CITE-expandspot { font-style : normal;\ncolor : green;\ncursor: hand;}\nDFN.collapsed { font-style : italic;\nfont-weight : normal;\ndisplay : 'none';\ncolor : red;}\n.mvd-DFN-collapsed { font-style : italic;\nfont-weight : normal;\ndisplay : 'none';\ncolor : red;}\nDFN.expanded { font-style : italic;\nfont-weight : normal;\ncolor : red;}\n.mvd-DFN-expanded { font-style : italic;\nfont-weight : normal;\ncolor : red;}\nEM.dropspot { cursor : hand;\ncolor : green;}\n.mvd-EM-dropspot { cursor : hand;\ncolor : green;}\n</style>\n<noscript><p class=\"Body\"><strong>JavaScript\n(active content) is\ndisabled. For all content to be accessible, you must enable JavaScripts\nin your browser.</strong></p>\n</noscript>\n\n<body style=\"background-color: rgb(255, 255, 255);\">", "<h1>", w73, w130, "Driver Readme</h1>\n<p class=\"Body\">" ("string"), "Month", w130, "Year", "<p class=\"Body\">To rate this instrument driver, go the the driver download page on the <a href=\"http://www.ni.com/idnet\">Instrument Driver Network</a>.</p> \n<p class=\"Body\">The readme contains the following main sections:</p>\n<ul>\n<li><a href=\"#Overview\">Overview</a></li>\n" ("string"), w156, w127, w154, w126, w152, w149, w145, w139, w138, w135, "</ul>\n" ("string"), w121, w117, w113, w109, w105, w101, w85, "<p class=\"Body\">Original Release Date: ", "OriginalReleaseDate", "</p>", "<p class=\"Body\">Current Revision Date: ", "CurrentRevisionDate", "</p><p></p>") -> (w124:string)
            }
            frame "Installation" {
              # "> Required Software >"
              # "> Installation >"
              n35 = local read "IsInstallation? chkBox"() -> (w176:bool)
              n36 = call "_2D array to HTML.vi"("Table (2D Array)"="Installation Instructions") -> ("HTML Code"=w172:string)  [unwired: 14 in]
              n37 = Concatenate Strings("<h2><a name=\"Installation\"></a>Installation</h2>\n<p class=\"Body\">This section documents installation\ninstructions for " ("string"), w162, " Instrument Driver.</p>\n<ol>" ("string"), w172, "</ol>\n" ("string")) -> (w170:string)
              n38 = Concatenate Strings("<h2><a name=\"RequiredSoft\"></a>Required Software</h2>\n<p class = \"Body\">Some software components need to be installed before using this instrument driver.\nThe minimum versions of these components are lised below.</p><p class=\"Body\">", "RequiredSoftware", "</p><p class=\"Body\">Refer to the <i>LabVIEW Help</i> for more information about software requirements.\n You access the <i>LabVIEW Help</i> by selecting <i>Help >> Search the LabVIEW Help</i></p>") -> (w163:string)
              n39 = Select(t=w170, s=w176, f="") -> (s? t:f=w168:string)
              n40 = Concatenate Strings(w169, w168, w163) -> (w167:string)
            }
            frame "Known Issues" {
              w182 = "<h2><a name = \"KnownIssues\"></a>Known Issues</h2>\n<p class = \"Body\">To report issues or provide feedback about this instrument driver,\nplease send and email to <a href=\"mailto:%s\">%s</a>.<p>%s</p>"  # <h2><a name = "KnownIssues"></a>Known Issues</h2> <p class = "Body">To report issues or provide feedback about this instrument driver, please send and email to <a href="mailto:%s">%s</a>.<p>%s</p>
              w185 = "<h2><a name=\"RevisionHistory\"></a>Revision History</h2>\n<p class = \"Body\">The latest version of this and other LabVIEW and LabWindows/CVI instrument drivers can be downloaded at the <a href=\"http://www.ni.com/idnet\">Instrument Driver Network</a>.</p><p class=\"Body\">%s</p>"  # <h2><a name="RevisionHistory"></a>Revision History</h2> <p class = "Body">The latest version of this and other LabVIEW and LabWindows/CVI instrument drivers can be downloaded at the <a href="http://www.ni.com/idnet">Instrument Driver Network</a>.</p><p class="Body">%s</p>
              n41 = Format Into String(format string=w182, "SupportEmail", "SupportEmail", "KnownIssues") -> (resulting string=w181:string)  [unwired: 2 in, 1 out]
              n42 = local read "IsKnownIssues? chkBox"() -> (w188:bool)
              n43 = Select(t=w181, s=w188, f="") -> (s? t:f=w189:string)
              n44 = Format Into String(format string=w185, "Revision History") -> (resulting string=w183:string)  [unwired: 2 in, 1 out]
              n45 = Concatenate Strings(w191, w189, w183) -> (w190:string)
            }
            frame "Developer" {
              n46 = Concatenate Strings("<a name=\"Developer\"></a>\n<h2>Developer(s) of " ("string"), w195, " Instrument Driver</h2>\n<p class=\"Body\">This instrument driver was developed by " ("string"), "AppDeveloper", "</p>\n<p class=\"Body\">Last upgrade of this instrument driver was made by " ("string"), "AppUpgrader", "</p>\n" ("string")) -> (w201:string)
              n47 = local read "IsDeveloper? chkBox"() -> (w203:bool)
              n48 = Select(t=w201, s=w203, f="") -> (s? t:f=w207:string)
              n49 = Concatenate Strings(w206, w207) -> (w205:string)
            }
            frame "Contact Support" {
              n50 = Concatenate Strings("<a name=\"Support\"></a>\n<h2>Contact Support</h2>\n<p class=\"Body\">You can contact our support staff by one\nof the following:</p>\n<p class=\"Body\"><span style=\"font-weight: bold;\">Telephone:&nbsp;</span>" ("string"), "SupportTelephone", "</p>\n<p class=\"Body\"><span style=\"font-weight: bold;\">Email:&nbsp;</span>" ("string"), "SupportEmail", "</p>\n<p class=\"Body\"><span style=\"font-weight: bold;\">Community\nForums:&nbsp;</span>" ("string"), "Support CommunityForums", "</p>\n<hr>" ("string")) -> (w219:string)
              n51 = local read "IsContactSupport? chkBox"() -> (w211:bool)
              n52 = Select(t=w219, s=w211, f="") -> (s? t:f=w222:string)
              n53 = Concatenate Strings(w221, w222) -> (w220:string)
            }
            frame "Copyright" {
              n54 = Concatenate Strings("<a name=\"Copyright\"></a>\n<h3><strong>Copyright</strong></h3>\n<p class=\"Body\">" ("string"), "Copyright", "</p>\n" ("string")) -> (w231:string)
              n55 = local read "IsCopyright? chkBox"() -> (w227:bool)
              n56 = Select(t=w231, s=w227, f="") -> (s? t:f=w234:string)
              n57 = Concatenate Strings(w233, w234) -> (w232:string)
            }
            frame "Trademarks" {
              n58 = Concatenate Strings("<a name=\"Trademarks\"></a>\n<h3><strong>Trademarks</strong></h3>\n<p class=\"Body\">" ("string"), "Trademarks", "</p>\n" ("string")) -> (w243:string)
              n59 = local read "IsTrademarks? chkBox"() -> (w242:bool)
              n60 = Select(t=w243, s=w242, f="") -> (s? t:f=w246:string)
              n61 = Concatenate Strings(w245, w246) -> (w244:string)
            }
            frame "Patents" {
              n62 = Concatenate Strings("<a name=\"Patents\"></a>\n<h3><strong>Patents</strong></h3>\n<p class=\"Body\">" ("string"), "Patents", "</p>\n" ("string")) -> (w253:string)
              n63 = local read "IsPatents? chkBox"() -> (w255:bool)
              n64 = Select(t=w253, s=w255, f="") -> (s? t:f=w258:string)
              n65 = Concatenate Strings(w257, w258) -> (w256:string)
            }
            frame "Disclaimer" {
              n66 = Concatenate Strings("<a name=\"Disclaimer\"></a>\n<h3><strong>Disclaimer</strong></h3>\n<p class=\"Body\">" ("string"), "Disclaimer", "\n</p>" ("string")) -> (w266:string)
              n67 = local read "IsDisclaimer? chkBox"() -> (w270:bool)
              n68 = Select(t=w266, s=w270, f="") -> (s? t:f=w273:string)
              n69 = Concatenate Strings(w269, w273, "</body></html>" ("string")) -> (w271:string)
            }
            frame "Shutdown" {
            }
          }
        }
        n70 = Write to Text File(file (use dialog)=w61, text=w60) -> (refnum out=w58:refnum<file>, error out=w59:errorcluster)  [unwired: 2 in, 1 out]
        n71 = Close File(refnum=w58, error in=w59) -> (error out=w54:errorcluster)  [unwired: 1 out]
      }
      frame "Shutdown" {
      }
    }
  }
  "HTML File Path" <- w6
  "error out" <- w1
